vi "Pose2D_parse.vi"(11 "字符串":string="5.77\"}, \"op\": \"publish\"}{\"topic\": \"/chatter\", \"msg\": {\"data\": \"hello world 1479387235.87\"}, \"op\": \"publish\"}{\"topic\": \"/chatter\", \"msg\": {\"data\": \"hello world 1479387235.97\"}, \"op\": \"publish\"}{\"topic\": \"/chatter\", \"msg\": {\"data\": \"hello world 1479387236.07\"}, \"op\": \"publish\"}{\"topic\": \"/chatter\", \"msg\": {\"data\": \"hello world 1479387236.17\"}, \"op\": \"publish\"}{\"topic\": \"/chatter\", \"msg\": {\"data\": \"hello world 1479387236.27\"}, \"op\": \"publish\"}{\"topic\": \"/chatter\", \"msg\": {\"data\": \"hello world 14793") -> (1 "theta":dbl, 2 "y":dbl, 3 "x":dbl)   [LabVIEW 2014]
panel:
  out "值":cluster{"x":dbl, "y":dbl, "theta":dbl}
  out "剩余字符串":string
  out "JSON out":string
  out "匹配之前的子字符串 2":string
  out "匹配+剩余字符串0":string
  out "匹配之前的子字符串":string
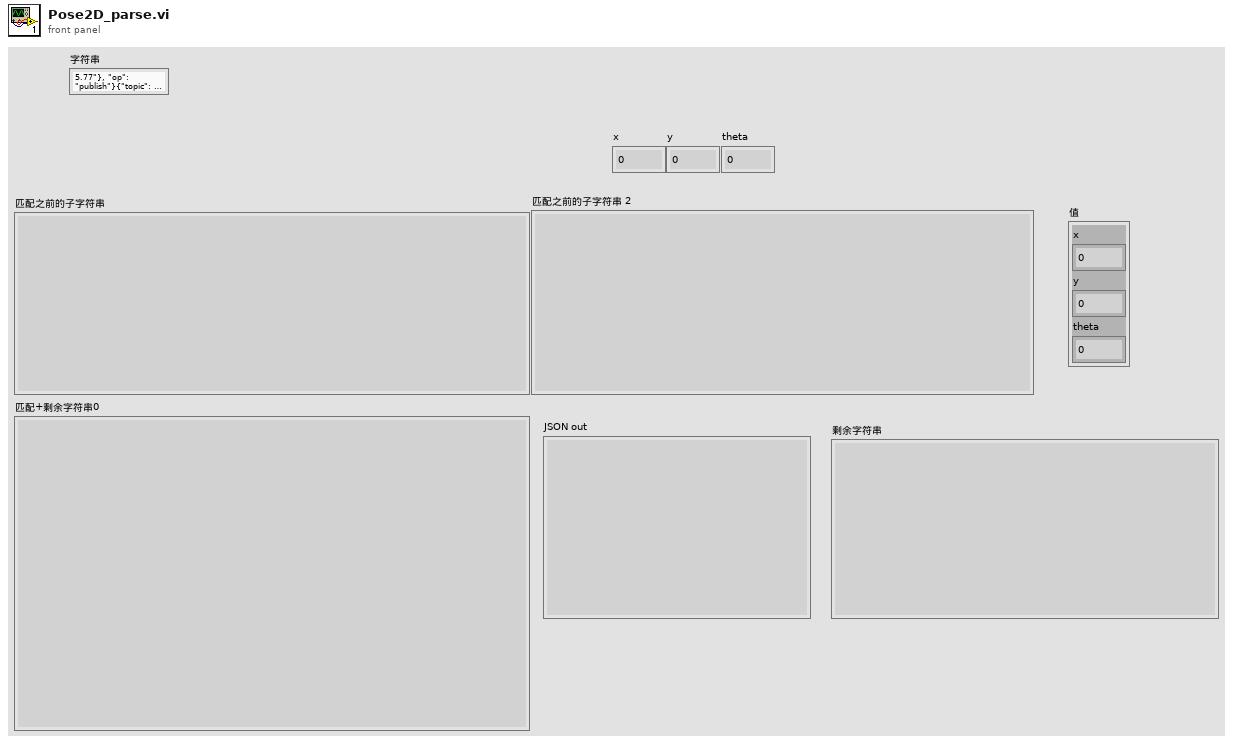
[diagram p1: front panel]
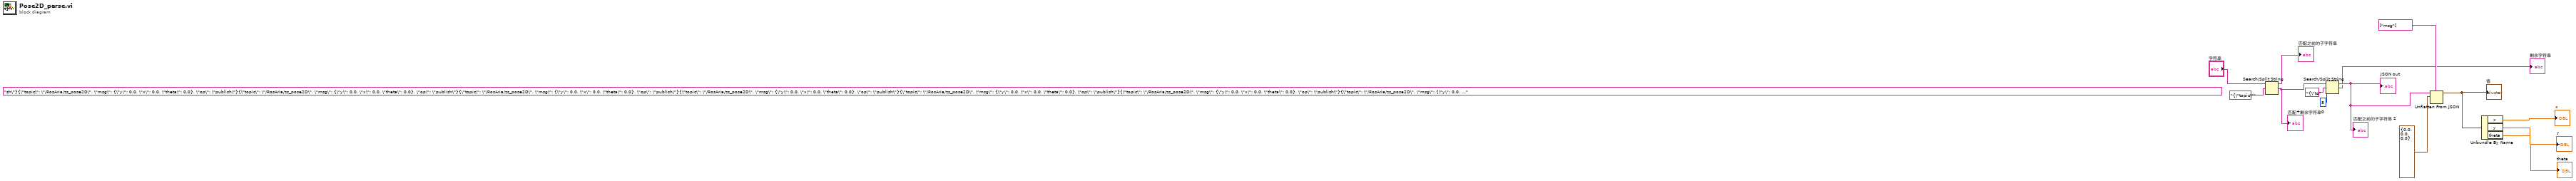
[diagram p0: block diagram]
diagram:
  (unwired) "sh\"}{\"topic\": \"/RosAria/zs_pose2D\", \"msg\": {\"y\": 0.0, \"x\": 0.0, \"theta\": 0.0}, \"op\": \"publish\"}{\"topic\": \"/RosAria/zs_pose2D\", \"msg\": {\"y\": 0.0, \"x\": 0.0, \"theta\": 0.0}, \"op\": \"publish\"}{\"topic\": \"/RosAria/zs_pose2D\", \"msg\": {\"y\": 0.0, \"x\": 0.0, \"theta\": 0.0}, \"op\": \"publish\"}{\"topic\": \"/RosAria/zs_pose2D\", \"msg\": {\"y\": 0.0, \"x\": 0.0, \"theta\": 0.0}, \"op\": \"publish\"}{\"topic\": \"/RosAria/zs_pose2D\", \"msg\": {\"y\": 0.0, \"x\": 0.0, \"theta\": 0.0}, \"op\": \"publish\"}{\"topic\": \"/RosAria/zs_pose2D\", \"msg\": {\"y\": 0.0, \"x\": 0.0, \"theta\": 0.0}, \"op\": \"publish\"}{\"topic\": \"/RosAria/zs_pose2D\", \"msg\": {\"y\": 0.0, \"x\": 0.0, \"theta\": 0.0}, \"op\": \"publish\"}{\"topic\": \"/RosAria/zs_pose2D\", \"msg\": {\"y\": 0.0, \"x\": 0.0, \"theta\": 0.0}, \"op\": \"publish\"}{\"topic\": \"/RosAria/zs_pose2D\", \"msg\": {\"y\": 0.0, \"x\": 0.0, \"theta\": 0.0}, \"op\": \"publish\"}{\"topic\": \"/RosAria/zs_pose2D\", \"msg\": {\"y\": 0.0, \"x\": 0.0, \"theta\": 0.0}, \"op\": \"publish\"}{\"topic\": \"/RosAria/zs_pose2D\", \"msg\": {\"y\": 0.0, \"x\": 0.0, \"theta\": 0.0}, \"op\": \"publ"
  n1 = Search/Split String(string="字符串", search string/char (-)="{\"topic\"" ("搜索字符串")) -> (substring before match=→"匹配之前的子字符串":string, match + rest of string=w5:string)  [unwired: 1 in, 1 out]
  "匹配+剩余字符串0" <- w5
  n2 = Search/Split String(string=w5, search string/char (-)="{\"to" ("搜索字符串/字符(-)"), offset (0)=8 ("偏移量(0)")) -> (substring before match=w12:string, match + rest of string=→"剩余字符串":string)  [unwired: 1 out]
  "匹配之前的子字符串 2" <- w12
  "JSON out" <- w12
  n3 = Unflatten From JSON(path=string[] ["msg"] ("路径"), JSON string=w12, type and defaults=cluster{"x":dbl, "y":dbl, "theta":dbl} {"x"=0.0, "y"=0.0, "theta"=0.0} ("类型和默认值")) -> (value=w9:cluster{"x":dbl, "y":dbl, "theta":dbl})  [unwired: 4 in, 1 out]
  "值" <- w9
  n4 = Unbundle By Name(w9) -> ("x"=→"x":dbl, "y"=→"y":dbl, "theta"=→"theta":dbl)
